vi "SubVI_Res_Init.vi"(8 "error in":errorcluster caption="에러 입력") -> (0 "error out":errorcluster caption="에러 출력", 3 "data":dynamicdata(graph) caption="데이터")   [LabVIEW 2016]
uses:
  <vilib>/DAQmx/read.llb/DAQmx Read.vi
  <vilib>/DAQmx/read.llb/DAQmx Read (Analog 1D Wfm NChan NSamp).vi
  <vilib>/DAQmx/create/channels.llb/DAQmx Create Channel (TEDS-AI-Voltage-Basic).vi
  <vilib>/DAQmx/create/channels.llb/DAQmx Create Channel (AI-Voltage-Basic).vi
  <vilib>/DAQmx/configure/timing.llb/DAQmx Timing (Sample Clock).vi
  <vilib>/DAQmx/miscellaneous.llb/DAQmx Fill In Error Info.vi
panel:
  out "task out":refnum<k21> caption="태스크 출력"
  in  "timeout (s)":dbl=10.0 caption="타임아웃(초)" format="%0.2f"
  in  "stop (T)":bool=TRUE caption="정지(T)"
  in  "속도":dbl=100000.0
  in  "샘플 개수":i32=2000
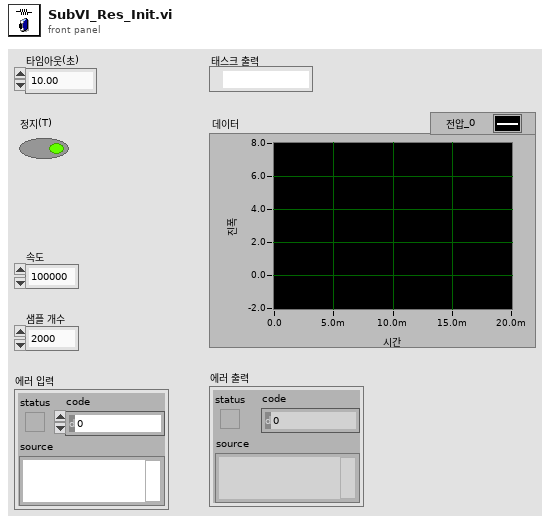
[diagram p1: front panel]
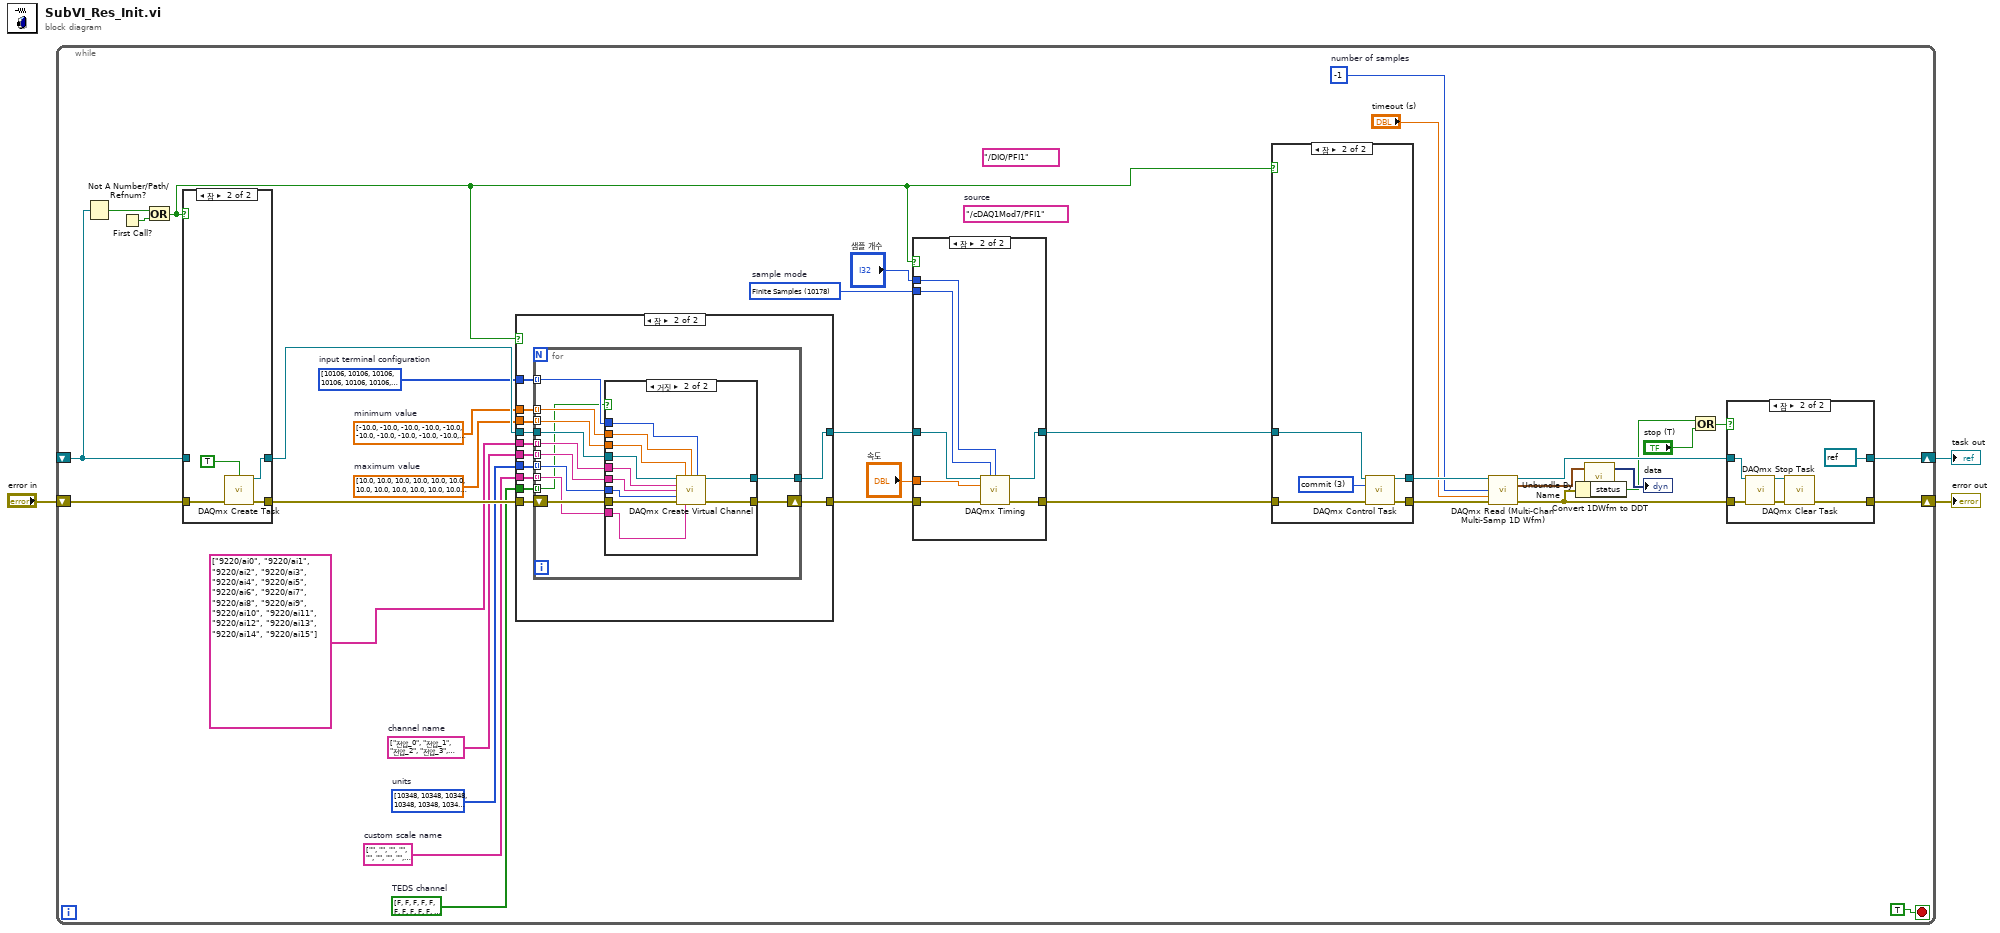
[diagram p0: block diagram]
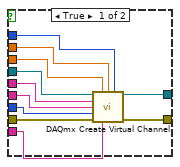
[diagram p6: hidden frame]
diagram:
  n1 = while {
    shift-right: [w12] -> w1
    shift-left: _ -> [w36]
    shift-right: [w10] -> w2
    shift-left: "error in" -> [w37]
    stop <- TRUE stop-if-true
    (unwired) tag "/DIO/PFI1" ("source")
    w16 = -1  # number of samples
    (unwired) "/cDAQ1Mod7/PFI1"  # source
    w20 = 10178 items=["Finite Samples"=10178, "Continuous Samples"=10123, "Hardware Timed Single Point"=12522]  # sample mode
    w25 = bool[] [FALSE, FALSE, FALSE, FALSE, FALSE, FALSE, FALSE, FALSE, FALSE, FALSE, FALSE, FALSE, FALSE, FALSE, FALSE, FALSE]  # TEDS channel
    w26 = string[] ["", "", "", "", "", "", "", "", "", "", "", "", "", "", "", ""]  # custom scale name
    w27 = i32[] [10348, 10348, 10348, 10348, 10348, 10348, 10348, 10348, 10348, 10348, 10348, 10348, 10348, 10348, 10348, 10348] items=["Volts"=10348, "From TEDS"=12516, "From Custom Scale"=10065]  # units
    w28 = string[] ["전압_0", "전압_1", "전압_2", "전압_3", "전압_4", "전압_5", "전압_6", "전압_7", "전압_8", "전압_9", "전압_10", "전압_11", "전압_12", "전압_13", "전압_14", "전압_15"]  # channel name
    w30 = dbl[] [10.0, 10.0, 10.0, 10.0, 10.0, 10.0, 10.0, 10.0, 10.0, 10.0, 10.0, 10.0, 10.0, 10.0, 10.0, 10.0]  # maximum value
    w31 = dbl[] [-10.0, -10.0, -10.0, -10.0, -10.0, -10.0, -10.0, -10.0, -10.0, -10.0, -10.0, -10.0, -10.0, -10.0, -10.0, -10.0]  # minimum value
    w32 = i32[] [10106, 10106, 10106, 10106, 10106, 10106, 10106, 10106, 10106, 10106, 10106, 10106, 10106, 10106, 10106, 10106] items=["default"=-1, "RSE"=10083, "NRSE"=10078, "Differential"=10106, "Pseudodifferential"=12529]  # input terminal configuration
    n2 = Not A Number/Path/Refnum?(number/path/refnum=w36) -> (NaN/Path/Refnum?=w35:bool)
    n3 = First Call?() -> (First Call?: T/F=w38:bool)
    n4 = Or(x=w35, y=w38) -> (x .or. y?=w19:bool)
    n5 = case "케이스 구조" shown="참" w19 {
      tunnel: [w113 w117] -> w34
      tunnel: w36 -> [w113 _]
      tunnel: [w112 w116] -> w33
      tunnel: w37 -> [w112 w114]
      frame False {
      }
      frame True {
        n6 = call <vilib>:"DAQmx Create Task.vi"("auto cleanup"=TRUE, "error in"=w114) -> ("task out"=w117:refnum<k21>, "error out"=w116:errorcluster)  [unwired: 12 in]
      }
    }
    n7 = case "케이스 구조" shown="참" w19 {
      tunnel: [w65 w75] -> w24
      tunnel: w34 -> [w65 w77]
      tunnel: [w64 w74] -> w23
      tunnel: w33 -> [w64 w76]
      tunnel: w32 -> [_ w73]
      tunnel: w31 -> [_ w72]
      tunnel: w30 -> [_ w71]
      tunnel: tag[] ["9220/ai0", "9220/ai1", "9220/ai2", "9220/ai3", "9220/ai4", "9220/ai5", "9220/ai6", "9220/ai7", "9220/ai8", "9220/ai9", "9220/ai10", "9220/ai11", "9220/ai12", "9220/ai13", "9220/ai14", "9220/ai15"] -> [_ w70]
      tunnel: w28 -> [_ w69]
      tunnel: w27 -> [_ w68]
      tunnel: w26 -> [_ w67]
      tunnel: w25 -> [_ w66]
      frame False {
      }
      frame True {
        n8 = for "For 루프" {
          tunnel: w77 -> [w89]
          tunnel: [w87] -> w75
          tunnel: w73 -> [w85] mode=indexing
          tunnel: w72 -> [w84] mode=indexing
          tunnel: w71 -> [w83] mode=indexing
          tunnel: w70 -> [w82] mode=indexing
          tunnel: w69 -> [w81] mode=indexing
          tunnel: w68 -> [w80] mode=indexing
          tunnel: w67 -> [w79] mode=indexing
          shift-right: [w86] -> w74
          shift-left: w76 -> [w88]
          tunnel: w66 -> [w78] mode=indexing
          n9 = case "케이스 구조" shown="거짓" w78 {
            tunnel: w89 -> [w100 w111]
            tunnel: w88 -> [w99 w110]
            tunnel: [w98 w109] -> w87
            tunnel: [w97 w108] -> w86
            tunnel: w85 -> [w96 w107]
            tunnel: w84 -> [w95 w106]
            tunnel: w83 -> [w94 w105]
            tunnel: w82 -> [w93 w104]
            tunnel: w81 -> [w92 w103]
            tunnel: w80 -> [w91 w102]
            tunnel: w79 -> [w90 w101]
            frame True {
              n10 = call-poly <vilib>:"DAQmx Create Virtual Channel.vi"("task in"=w100, "maximum value"=w94, "minimum value"=w95, "input terminal configuration"=w96, "physical channels"=w93, "name to assign"=w92, "units"=w91, "error in"=w99, "custom scale name"=w90) -> ("task out"=w98:refnum<k21>, "error out"=w97:errorcluster)  [unwired: 5 in]
            }
            frame False {
              n11 = call-poly <vilib>:"DAQmx Create Virtual Channel.vi"("task in"=w111, "maximum value"=w105, "minimum value"=w106, "input terminal configuration"=w107, "physical channels"=w104, "name to assign"=w103, "units"=w102, "error in"=w110, "custom scale name"=w101) -> ("task out"=w109:refnum<k21>, "error out"=w108:errorcluster)  [unwired: 5 in]
            }
          }
        }
      }
    }
    n12 = case "케이스 구조" shown="참" w19 {
      tunnel: [w56 w58] -> w4
      tunnel: w24 -> [w56 w61]
      tunnel: [w55 w57] -> w5
      tunnel: w23 -> [w55 w59]
      tunnel: "샘플 개수" -> [_ w63]
      tunnel: w20 -> [_ w62]
      tunnel: "속도" -> [_ w60]
      frame False {
      }
      frame True {
        n13 = call-poly <vilib>:"DAQmx Timing.vi"("task/channels in"=w61, "sample mode"=w62, "samples per channel"=w63, "rate"=w60, "error in"=w59) -> ("task out"=w58:refnum<k21>, "error out"=w57:errorcluster)  [unwired: 9 in]
      }
    }
    n14 = case "케이스 구조" shown="참" w19 {
      tunnel: [w49 w53] -> w18
      tunnel: w4 -> [w49 w54]
      tunnel: [w48 w51] -> w17
      tunnel: w5 -> [w48 w52]
      frame False {
      }
      frame True {
        w50 = 3 items=["verify"=2, "reserve"=4, "commit"=3, "unreserve"=5, "abort"=6] ("action")
        n15 = call <vilib>:"DAQmx Control Task.vi"("task/channels in"=w54, "action"=w50, "error in"=w52) -> ("task out"=w53:refnum<k21>, "error out"=w51:errorcluster)  [unwired: 11 in]
      }
    }
    n16 = call-poly "DAQmx Read (Multi-Chan Multi-Samp 1D Wfm).vi"("task/channels in"=w18, "number of samples per channel"=w16, "timeout"="timeout (s)", "error in"=w17) -> ("task out"=w11:refnum<k21>, "data"=w15:waveform(dbl)[], "error out"=w9:errorcluster)  [unwired: 9 in]
    n17 = Unbundle By Name(w9) -> ("status"=w8:bool)
    n18 = call <vilib>:"Convert 1DWfm to DDT.vi"("Array of Waveforms"=w15) -> ("Dynamic Data Type"=→"data":dynamicdata)  [unwired: 3 in]
    n19 = Or(x=w8, y="stop (T)") -> (x .or. y?=w6:bool)
    n20 = case "케이스 구조" shown="참" w6 {
      tunnel: [w41 refnum<k21> refnum ("task in")] -> w12
      tunnel: w11 -> [w41 w47]
      tunnel: [w40 w44] -> w10
      tunnel: w9 -> [w40 w46]
      frame False {
      }
      frame True {
        n21 = call <vilib>:"DAQmx Stop Task.vi"("task/channels in"=w47, "error in"=w46) -> ("task out"=w43:refnum<k21>, "error out"=w45:errorcluster)  [unwired: 12 in]
        n22 = call <vilib>:"DAQmx Clear Task.vi"("task in"=w43, "error in"=w45) -> ("error out"=w44:errorcluster)  [unwired: 13 in]
      }
    }
  }
  "error out" <- w2
  "task out" <- w1
